vi "init.vi"(8 "error in":errorcluster, 10 "tree control reference":refnum<k24>, 11 "tree_control in":refnum<class "vs_tree_control.lvclass">) -> (0 "error out":errorcluster, 3 "tree_control out":refnum<class "vs_tree_control.lvclass">)   [LabVIEW 2020, in "vs_tree_control.lvclass"]
uses:
  vs_tree_control.lvclass
  vs_tree_control.lvclass/vs_tree_control.ctl
  NationalInstruments.VeriStand.SystemStorageUI
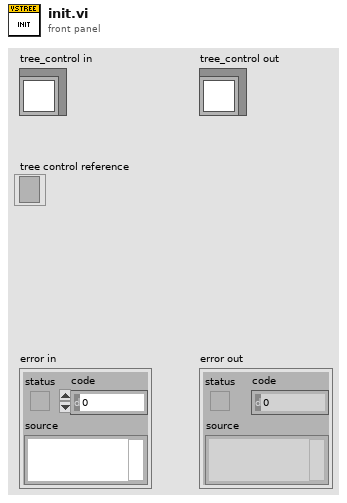
[diagram p1: front panel]
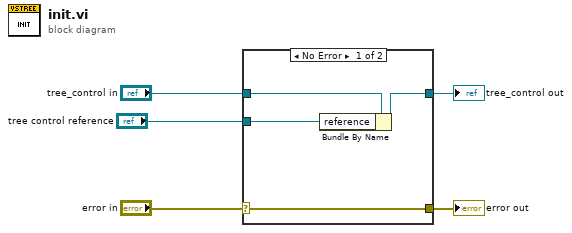
[diagram p0: block diagram]
diagram:
  n1 = case shown="No Error" "error in" {
    selector: "error in" -> [w6 w11]
    tunnel: [w6 w11] -> w4
    tunnel: [w8 w10] -> w2
    tunnel: "tree_control in" -> [w9 w10]
    tunnel: "tree control reference" -> [w7 _]
    frame No Error {
      n2 = Bundle By Name(cluster=w9, "reference"=w7) -> (w8:refnum<class "vs_tree_control.lvclass">)
    }
    frame Error {
    }
  }
  "error out" <- w4
  "tree_control out" <- w2
